vi "Test_Benchmarking_LocalLogValueEventTypeBoolCall_AvgCallTimeSub10uS.vi"(8 "error in (no error)":errorcluster, 11 "Benchmarking in":refnum<class "Benchmarking.lvclass">) -> (0 "error out":errorcluster, 3 "Benchmarking out":refnum<class "Benchmarking.lvclass">)   [LabVIEW 2017, in "Benchmarking.lvclass"]
uses:
  Benchmarking.lvclass
  Source/Composed Log/LoggerReference/LoggerReference.lvclass/LoggerReference.ctl
  Source/Composed Log/Types/Log Level.ctl
  c732dfe6-6ae6-40e1-b7d0-4452a78b430e.vi
  3a172113-d25b-462f-a03e-81be6615e529.vi
  <vilib>/Analysis/baseanly.llb/Mean (DBL).vi
  Source/Composed Log/LoggerReference/Return Aggregate Queues.vi
  Source/Composed Log/LoggerReference/Add Aggregate Log.vi
  c732dfe6-6ae6-40e1-b7d0-4452a78b430e.vi/cf67eb2b-dd56-49d4-9907-15017b47e902.vi
  3a172113-d25b-462f-a03e-81be6615e529.vi/a5f216a8-0110-4e40-abef-7258c7e6fa36.vi
  Source/Composed Log/LoggerReference/Log Event.vi
  Source/Composed Log/LoggerReference/Send Add Sink.vi
  Source/Composed Log/LoggerReference/Log.vi
  Source/Composed Log/LoggerReference/Remove Stale Logs.vi
  Source/LVQueue Sink/LVQueue Sink.lvclass
  C:/CS/Internal/LabVIEW/Logger/Source/Composed Log/Log Sink/Log Sink.lvclass
  Source/Composed Log/Application Logger/Launch Worker Loop.vi
  Source/Composed Log/LoggerReference/Initialize Logger Instance.vi
  Source/Composed Log/LoggerReference/LoggerReference.lvclass
  Source/Composed Log/IErrorFormat/IErrorFormat.lvclass
  Source/Composed Log/Log Sink/Log Sink.lvclass
  Source/Composed Log/Composed Log.lvlib
  <vilib>/Analysis/NI_AALBase.lvlib
  <vilib>/addons/_JKI Toolkits/VI Tester/TestCase.llb/TestCase.lvclass
  C:/Program Files (x86)/National Instruments/LabVIEW 2017/vi.lib/addons/_JKI Toolkits/VI Tester/TestCase.llb/TestCase.lvclass
panel:
  in  "Numeric":i32=10000
  out "min index(es)":i32
  out "max index(es)":i32
  out "Histogram Graph":T1(graph)
  out "Benchmark Results":string
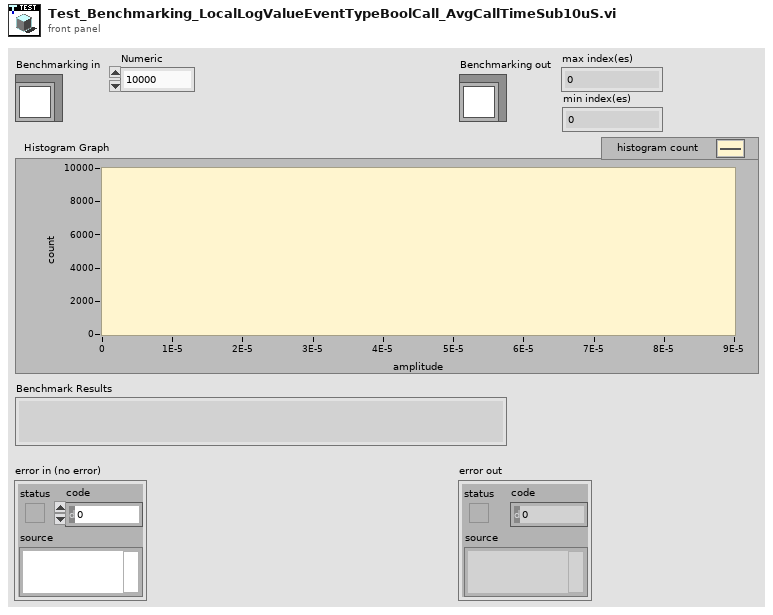
[diagram p1: front panel]
types:
  T1 = cluster{"X Values":dbl[], "Histogram: h(x)":i32[]}
  T2 = typedef "Composed Log.lvlib/Log Level.ctl" = enum16{"Debug", "Info", "Warning", "Error", "Critical"}
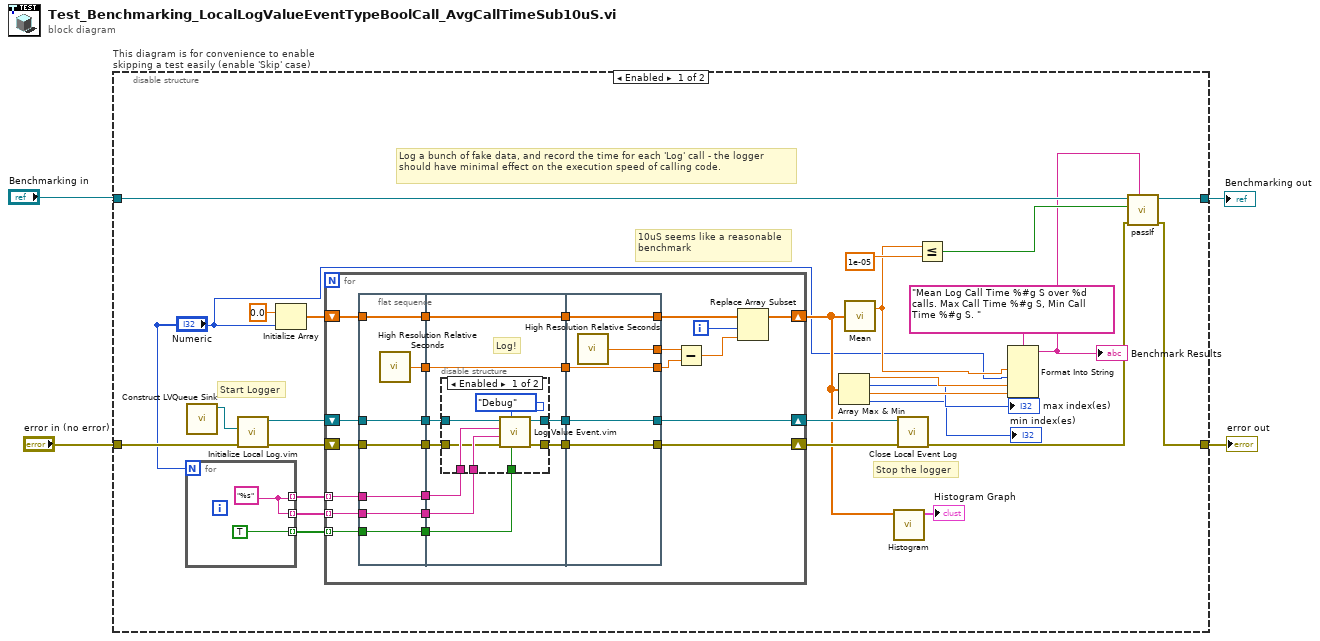
[diagram p0: block diagram]
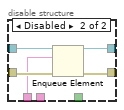
[diagram p2: hidden frame]
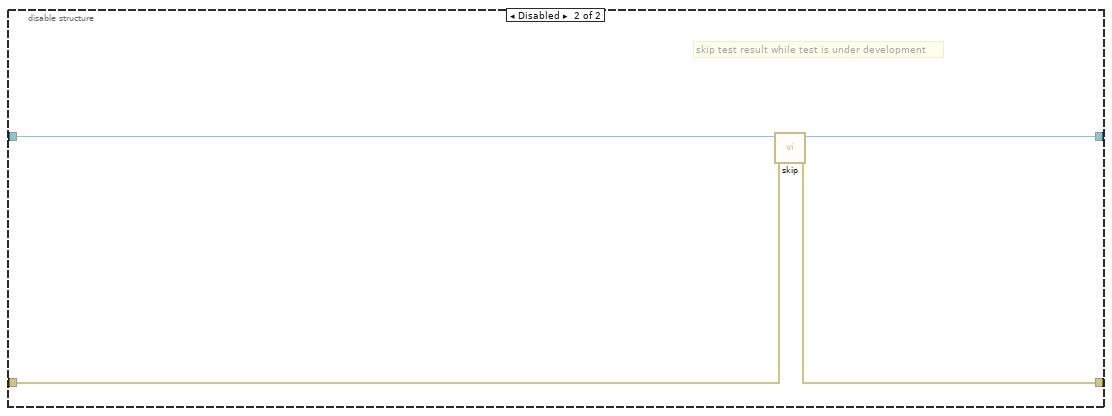
[diagram p3: hidden frame]
diagram:
  n1 = disable-structure "This diagram is for convenience to enable skipping a test easily (enable 'Skip' case)" shown="Enabled" {
    disable-tunnel: "Benchmarking in" -> [w27 w96]
    disable-tunnel: [w26 w94] -> w4
    disable-tunnel: [w28 w95] -> w3
    disable-tunnel: "error in (no error)" -> [w16 w93]
    frame Enabled {
      # "Stop the logger"
      # "10uS seems like a reasonable    benchmark"
      # "Start Logger"
      # "Log a bunch of fake data, and record the time for each 'Log' call - the logger should have minimal effect on the execution speed of calling code."
      n2 = for {
        N: "Numeric" -> [_]
        tunnel: [w92] -> w31 mode=indexing
        tunnel: [w92] -> w25 mode=indexing
        tunnel: [TRUE] -> w5 mode=indexing
        w92 = "%s"
      }
      n3 = call "Construct LVQueue Sink.vi"() -> ("LVQueue Sink out"=w14:refnum<class "LVQueue Sink.lvclass">)  [unwired: 10 in, 1 out]
      n4 = call "Initialize Local Log.vim"("error in (no error)"=w16, "Startup Sink(s)"=w14) -> ("error out"=w15:errorcluster, "Log Instance Reference"=w13:refnum<class "LoggerReference.lvclass">)  [unwired: 7 in, 1 out]
      n5 = Initialize Array(0.0 ("element"), "Numeric") -> (w29:dbl[])
      n6 = for {
        tunnel: w31 -> [w51] mode=indexing
        shift-right: [w49] -> w18
        shift-left: w15 -> [w50]
        shift-right: [w40] -> w11
        shift-left: w29 -> [w46]
        tunnel: w25 -> [w39] mode=indexing
        shift-right: [w34] -> w12
        shift-left: w13 -> [w36]
        tunnel: w5 -> [w33] mode=indexing
        i -> [w42]
        n7 = flat-sequence {
          tunnel: w50 -> [w62]
          tunnel: w51 -> [w63]
          tunnel: [w63] -> w56
          tunnel: [w62] -> w55
          tunnel: [w61] -> w54
          tunnel: w46 -> [w60]
          tunnel: [w60] -> w44
          tunnel: w39 -> [w59]
          tunnel: [w59] -> w38
          tunnel: [w58] -> w37
          tunnel: w36 -> [w58]
          tunnel: w33 -> [w57]
          tunnel: [w57] -> w32
          tunnel: w56 -> [w68]
          tunnel: w55 -> [w72]
          tunnel: w54 -> [w70]
          tunnel: [w71] -> w53
          tunnel: [w70] -> w52
          tunnel: [w69] -> w45
          tunnel: w44 -> [w69]
          tunnel: w38 -> [w67]
          tunnel: w37 -> [w66]
          tunnel: [w65] -> w35
          tunnel: w32 -> [w64]
          tunnel: [w89] -> w48
          tunnel: [w90] -> w49
          tunnel: w53 -> [w90]
          tunnel: w52 -> [w89]
          tunnel: [w88] -> w47
          tunnel: [w87] -> w43
          tunnel: w45 -> [w87]
          tunnel: w35 -> [w86]
          tunnel: [w86] -> w34
          frame #0 {
            n8 = call <vilib>:"High Resolution Relative Seconds.vi"() -> ("relative seconds"=w61:dbl)
          }
          frame #1 {
            # "Log!"
            n9 = disable-structure shown="Enabled" {
              disable-tunnel: w72 -> [w75 w84]
              disable-tunnel: [w76 w83] -> w71
              disable-tunnel: w68 -> [w79 w81]
              disable-tunnel: w67 -> [w78 _]
              disable-tunnel: w66 -> [w80 w85]
              disable-tunnel: [w77 w85] -> w65
              disable-tunnel: w64 -> [w74 _]
              frame Enabled {
                n10 = call "Log Value Event.vim"("Value(s)"=w74, "Event Level"=Log_Level."Debug", "error in (no error)"=w75, "Log Message Format String"=w78, "Event Source"=w79, "LoggerReference in"=w80) -> ("error out"=w76:errorcluster, "LoggerReference out"=w77:refnum<class "LoggerReference.lvclass">)  [unwired: 4 in]
              }
              frame Disabled {
                n11 = Enqueue Element(element=w81, error in (no error)=w84) -> (queue=w82:refnum<queue>, error out=w83:errorcluster)  [unwired: 1 in, 2 out]
              }
            }
          }
          frame #2 {
            n12 = call <vilib>:"High Resolution Relative Seconds.vi"() -> ("relative seconds"=w88:dbl)
          }
        }
        n13 = Subtract(x=w47, y=w48) -> (x-y=w41:dbl)
        n14 = Replace Array Subset(array=w43, new element=w41, index=w42) -> (w40:dbl[])
      }
      n15 = Array Max & Min(array=w11) -> (max value=w21:dbl, max index (indices)=→"max index(es)":i32, min value=w20:dbl, min index (indices)=→"min index(es)":i32)
      n16 = call-poly <vilib>:"Mean.vi"("X"=w11) -> ("mean"=w7:dbl)  [unwired: 1 out]
      n17 = call <vilib>:"Histogram.vi"("X"=w11) -> ("Histogram Graph"=→"Histogram Graph":T1)  [unwired: 7 in, 3 out]
      n18 = call "Close Local Event Log.vi"("error in (no error)"=w18, "Log Instance"=w12) -> ("error out"=w17:errorcluster)  [unwired: 9 in]
      n19 = Less Or Equal?(x=w7, y=1e-05) -> (x <= y?=w23:bool)
      n20 = Format Into String(format string="Mean Log Call Time %#g S over %d calls. Max Call Time %#g S, Min Call Time %#g S. ", w7, "Numeric", w21, w20) -> (resulting string=w19:string)  [unwired: 2 in, 1 out]
      "Benchmark Results" <- w19
      n21 = call-dynamic "passIf.vi"("custom report message (\"\")"=w19, "error in (no error)"=w17, "pass"=w23, "TestCase in"=w27) -> ("error out"=w28:errorcluster, "TestCase out"=w26:refnum<class "Benchmarking.lvclass">)  [unwired: 6 in]
    }
    frame Disabled {
      # "skip test result while test is under development"
      n22 = call <vilib>:"skip.vi"("error in (no error)"=w93, "TestCase in"=w96) -> ("error out"=w95:errorcluster, "TestCase out"=w94:refnum<class "Benchmarking.lvclass">)  [unwired: 8 in]
    }
  }
  "error out" <- w3
  "Benchmarking out" <- w4
